vi "MaxEye_ATE_Load Configuration_Extract Value From Header.vi"(9 "Label Name":string, 10 "Class Name":string, 11 "File Data in":string) -> (1 "File Data Remaining":string, 3 "File Data out":string)   [LabVIEW 2021]
panel:
  out "offset past match":i32
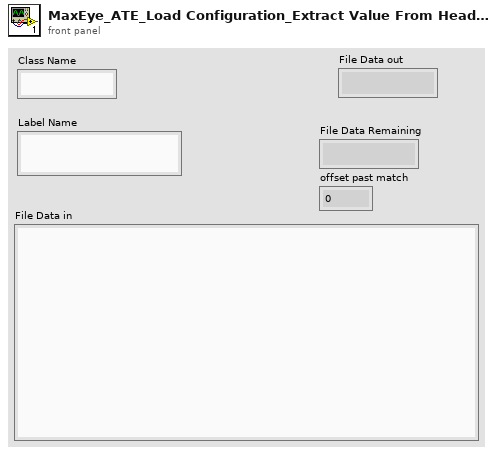
[diagram p1: front panel]
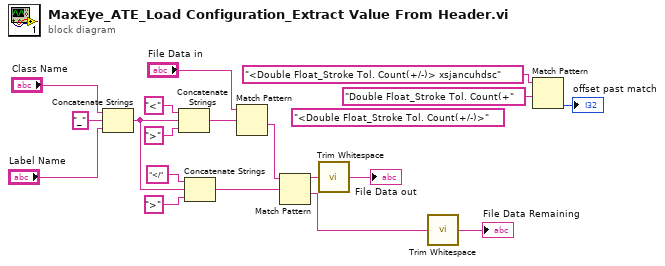
[diagram p0: block diagram]
diagram:
  (unwired) "<Double Float_Stroke Tol. Count(+/-)>" ("regular expression")
  n1 = Concatenate Strings("Class Name", "_" ("string"), "Label Name") -> (w12:string)
  n2 = Concatenate Strings("<" ("string"), w12, ">" ("string")) -> (w1:string)
  n3 = Concatenate Strings("</" ("string"), w12, ">" ("string")) -> (w9:string)
  n4 = Match Pattern(string="File Data in", regular expression=w1) -> (after substring=w18:string)  [unwired: 1 in, 3 out]
  n5 = Match Pattern(string=w18, regular expression=w9) -> (before substring=w19:string, after substring=w8:string)  [unwired: 1 in, 2 out]
  n6 = call <vilib>:"Trim Whitespace.vi"("string"=w19) -> ("trimmed string"=→"File Data out":string)  [unwired: 1 in]
  n7 = call <vilib>:"Trim Whitespace.vi"("string"=w8) -> ("trimmed string"=→"File Data Remaining":string)  [unwired: 1 in]
  n8 = Match Pattern(string="<Double Float_Stroke Tol. Count(+/-)> xsjancuhdsc", regular expression="Double Float_Stroke Tol. Count(+" ("string")) -> (offset past match=→"offset past match":i32)  [unwired: 1 in, 3 out]
